vi "getMetaData_withAvg_TF.vi"(10 "MetaDataPath":path) -> (0 "Num Samples":i32[](array[numeric]), 1 "freqs (hz)":dbl[](array[numeric]), 2 "ControlParams":T1)   [LabVIEW 2017]
uses:
  sysID_ControlParams.ctl
  <vilib>/Utility/file.llb/Read From Spreadsheet File (DBL).vi
panel:
  out "all rows":dbl[][](array[numeric]) format="%0.3f"
  out "Ts (from meta_data.csv)":dbl=1.0
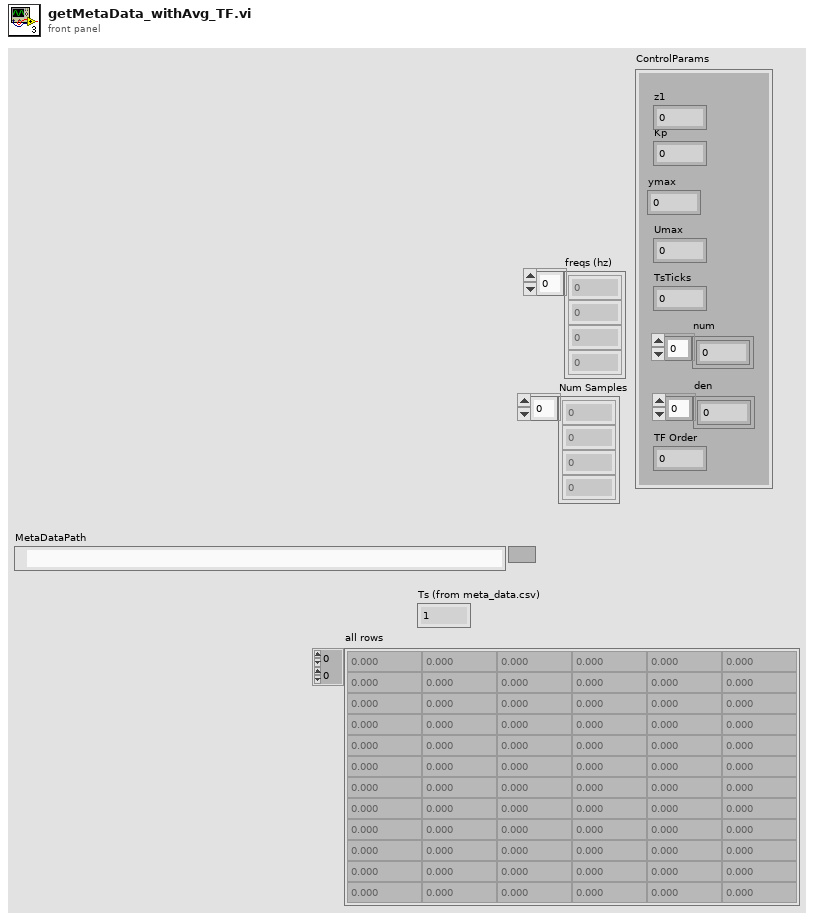
[diagram p1: front panel]
types:
  T1 = typedef "sysID_ControlParams.ctl" = cluster{"Kp":sgl, "Umax ":sgl, "ymax":sgl, "TsTicks":u32, "z1":sgl, "num":sgl[], "den":sgl[], "TF Order":u8}
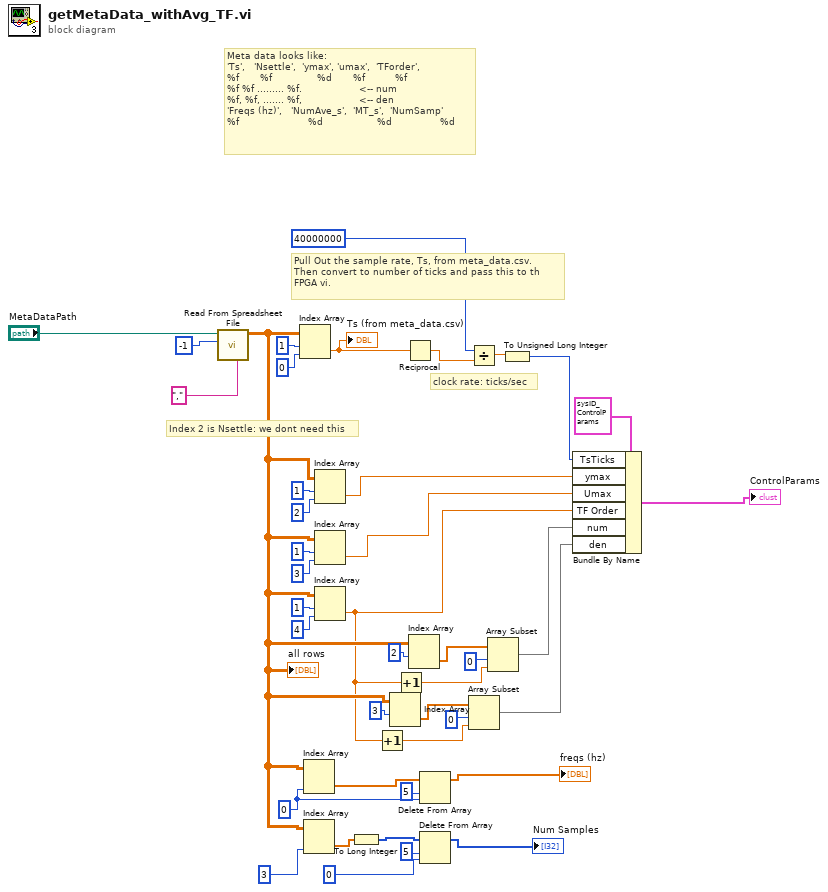
[diagram p0: block diagram]
diagram:
  w27 = 0
  # "Meta data looks like:\n'Ts',   'Nsettle',  'ymax', 'umax',  'TForder',\n%f       %f               %d       %f          %f\n%f %f ......... %f.                   <-- num\n%f, %f, ....... %f,                   <-- den      \n'Freqs (hz)',   'NumAve_s',  'MT_s',  'NumSamp'\n%f                       %d                  %d                %d"
  # "Index 2 is Nsettle: we dont need this"
  # "clock rate: ticks/sec"
  # "Pull Out the sample rate, Ts, from meta_data.csv.\nThen convert to number of ticks and pass this to th\nFPGA vi."
  n1 = call-poly <vilib>:"Read From Spreadsheet File.vi"("delimiter (\\t)"=",", "number of rows (all:-1)"=-1, "file path (dialog if empty)"="MetaDataPath") -> ("all rows"=w5:dbl[][])  [unwired: 4 in, 4 out]
  "all rows" <- w5
  n2 = Index Array(array=w5, index (row)=1, index (col)=0) -> (element=w42:dbl)
  "Ts (from meta_data.csv)" <- w42
  n3 = Index Array(array=w5, index (col)=w27) -> (element=w28:dbl[])  [unwired: 1 in]
  n4 = Index Array(array=w5, index (col)=3) -> (element=w17:dbl[])  [unwired: 1 in]
  n5 = Index Array(array=w5, index (row)=1, index (col)=2) -> (element=w30:dbl)
  n6 = Index Array(array=w5, index (row)=1, index (col)=3) -> (element=w29:dbl)
  n7 = Index Array(array=w5, index (row)=1, index (col)=4) -> (element=w4:dbl)
  n8 = To Long Integer(number=w17) -> (32bit integer=w18:i32[])
  n9 = Increment(x=w4) -> (x+1=w6:dbl)
  n10 = Index Array(array=w5, index (row)=3) -> (element=w8:dbl[])  [unwired: 1 in]
  n11 = Increment(x=w4) -> (x+1=w10:dbl)
  n12 = Reciprocal(x=w42) -> (1/x=w39:dbl)
  n13 = Index Array(array=w5, index (row)=2) -> (element=w13:dbl[])  [unwired: 1 in]
  n14 = Delete From Array(array=w28, length=5, index=w27) -> (array with subset deleted=→"freqs (hz)":dbl[])  [unwired: 1 out]
  n15 = Delete From Array(array=w18, length=5, index=0) -> (array with subset deleted=→"Num Samples":i32[])  [unwired: 1 out]
  n16 = Divide(x=40000000, y=w39) -> (x/y=w41:dbl)
  n17 = Array Subset(array=w8, index=0, length=w6) -> (w3:dbl[])
  n18 = Array Subset(array=w13, index=0, length=w10) -> (w11:dbl[])
  n19 = To Unsigned Long Integer(number=w41) -> (unsigned 32bit integer=w24:u32)
  n20 = Bundle By Name(cluster=T1 {"Kp"=0.0, "Umax "=0.0, "ymax"=0.0, "TsTicks"=0, "z1"=0.0, "num"=[0.0, 0.0, 0.0, 0.0, 0.0, 0.0, 0.0, 0.0, 0.0], "den"=[0.0, 0.0, 0.0, 0.0, 0.0, 0.0, 0.0, 0.0, 0.0], "TF Order"=0} ("ControlParams"), "TsTicks"=w24, "ymax"=w30, "Umax"=w29, "TF Order"=w4, "num"=w11, "den"=w3) -> (→"ControlParams":T1)
